vi "get cipher information.vi"(8 "error in":errorcluster, 11 "cipher name":string) -> (0 "error out":errorcluster, 2 "sizes":T1)   [LabVIEW 2016, in "lvlibcrypto cipher.lvclass"]
doc: "EVP_enc_null()\nNull cipher: does nothing.\n \n \nEVP_aes_128_cbc(), EVP_aes_128_ecb(), EVP_aes_128_cfb(), EVP_aes_128_ofb()\nAES with a 128-bit key in CBC, ECB, CFB and OFB modes respectively.\n \n \nEVP_aes_192_cbc(), EVP_aes_192_ecb(), EVP_aes_192_cfb(), EVP_aes_192_ofb()\nAES with a 192-bit key in CBC, ECB, CFB and OFB modes respectively.\n \n \nEVP_aes_256_cbc(), EVP_aes_256_ecb(), EVP_aes_256_cfb(), EVP_aes_256_ofb()\nAES with a 256-bit key in CBC, ECB, CFB and OFB modes respectively.\n \n \nEVP_des_cbc(), EVP_des_ecb(), EVP_des_cfb(), EVP_des_ofb()\nDES in CBC, ECB, CFB and OFB modes respectively.\n \n \nEVP_des_ede_cbc(), EVP_des_ede(), EVP_des_ede_ofb(), EVP_des_ede_cfb()\nTwo key triple DES in CBC, ECB, CFB and OFB modes respectively.\n \n \nEVP_des_ede3_cbc(), EVP_des_ede3(), EVP_des_ede3_ofb(), EVP_des_ede3_cfb()\nThree key triple DES in CBC, ECB, CFB and OFB modes respectively.\n \n \nEVP_desx_cbc()\nDESX algorithm in CBC mode.\n \n \nEVP_rc4()\nRC4 stream cipher. This is a variable key length cipher with default key length 128 bits.\n \n \nEVP_rc4_40()\nRC4 stream cipher with 40-bit key length. This is obsolete and new code should use EVP_rc4() and the EVP_CIPHER_CTX_set_key_length() function.\n \n \nEVP_idea_cbc(), EVP_idea_ecb(), EVP_idea_cfb(), EVP_idea_ofb()\nIDEA encryption algorithm in CBC, ECB, CFB and OFB modes respectively.\n \n \nEVP_rc2_cbc(), EVP_rc2_ecb(), EVP_rc2_cfb(), EVP_rc2_ofb()\nRC2 encryption algorithm in CBC, ECB, CFB and OFB modes respectively. This is a variable key length cipher with an additional parameter called \"effective key bits\" or \"effective key length\". By default both are set to 128 bits.\n \n \nEVP_rc2_40_cbc(), EVP_rc2_64_cbc()\nRC2 algorithm in CBC mode with a default key length and effective key length of 40 and 64 bits. These are obsolete and new code should use EVP_rc2_cbc(), EVP_CIPHER_CTX_set_key_length(), and EVP_CIPHER_CTX_ctrl() to set the key length and effective key length.\n \n \nEVP_bf_cbc(), EVP_bf_ecb(), EVP_bf_cfb(), EVP_bf_ofb()\nBlowfish encryption algorithm in CBC, ECB, CFB and OFB modes respectively. This is a variable key length cipher.\n \n \nEVP_cast5_cbc(), EVP_cast5_ecb(), EVP_cast5_cfb(), EVP_cast5_ofb()\nCAST encryption algorithm in CBC, ECB, CFB and OFB modes respectively. This is a variable key length cipher.\n \n \nEVP_rc5_32_12_16_cbc(), EVP_rc5_32_12_16_ecb(), EVP_rc5_32_12_16_cfb(), EVP_rc5_32_12_16_ofb()\nRC5 encryption algorithm in CBC, ECB, CFB and OFB modes respectively. This is a variable key length cipher with an additional \"number of rounds\" parameter. By default the key length is set to 128 bits and 12 rounds.\n \n \nEVP_aes_128_gcm(), EVP_aes_192_gcm(), EVP_aes_256_gcm()\nAES Galois Counter Mode (GCM) for 128, 192 and 256 bit keys respectively. These ciphers require additional control operations to function correctly: see the GCM mode section below for details.\n \n \nEVP_aes_128_ccm(), EVP_aes_192_ccm(), EVP_aes_256_ccm()\nAES Counter with CBC-MAC Mode (CCM) for 128, 192 and 256 bit keys respectively. These ciphers require additional control operations to function correctly: see CCM mode section below for details.\n \n \nEVP_chacha20()\nThe ChaCha20 stream cipher. The key length is 256 bits, the IV is 96 bits long."
uses:
  lvlibcrypto cipher.lvclass
  tls library paths.vi
  add all ciphers.vi
  <vilib>/Utility/error.llb/Error Cluster From Error Code.vi
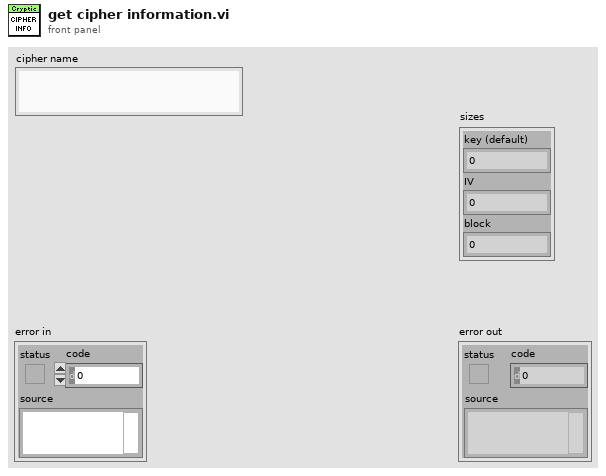
[diagram p1: front panel]
types:
  T1 = cluster{"key (default)":i32, "IV":i32, "block":i32}
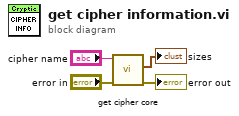
[diagram p0: block diagram]
diagram:
  n1 = call "get cipher core.vi"("error in"="error in", "cipher name"="cipher name") -> ("error out"=→"error out":errorcluster, "sizes"=→"sizes":T1)  [unwired: 7 in, 1 out]
